vi "RSZVB Send Channel Trigger and Wait for OPC.vi"(8 "error in (no error)":errorcluster, 9 "Timeout (15000)":i32=15000, 10 "Channel (1)":i32=1, 11 "VISA session":refnum<visa-resource-name>) -> (0 "error out":errorcluster {"code" format="%.0x"}, 3 "dup VISA session":refnum<visa-resource-name>)   [LabVIEW 2015]
doc: "This VI starts a new single sweep sequence and waits for operation completed (OPC) before returning the status code. This function is available in single sweep mode only (INITiate<Ch>:CONTinuous OFF).\n\nNote(s):\n\n(1) In contrast to all other functions of the analyzer, INITiate<Ch>[:IMMediate] has been implemented to prevent overlapped execution.\n\n(2) The data of the last sweep can be read using CALCulate<Ch>:DATA:NSWeep? SDATa, <history_count>.\n\nRemote-control command(s):\nINITiate<Ch>[:IMMediate]\n*OPC?"
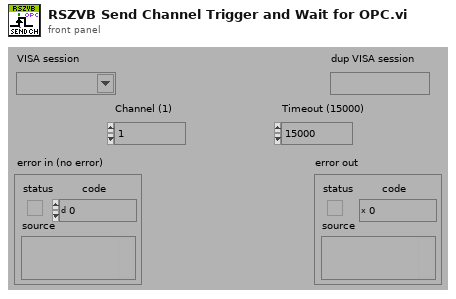
[diagram p1: front panel]
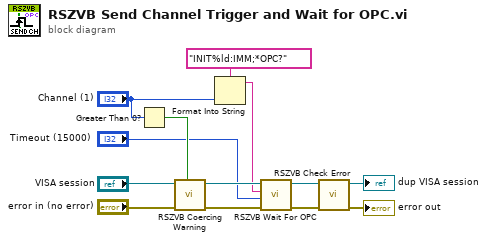
[diagram p0: block diagram]
diagram:
  n1 = Greater Than 0?(x="Channel (1)") -> (x > 0?=w6:bool)
  n2 = call "RSZVB Coercing Warning.vi"("In Range?"=w6, "error in (no error)"="error in (no error)", "VISA session"="VISA session") -> ("error out"=w9:errorcluster, "dup VISA session"=w10:refnum<visa-resource-name>)  [unwired: 7 in]
  n3 = Format Into String(format string="INIT%ld:IMM;*OPC?", "Channel (1)") -> (resulting string=w8:string)  [unwired: 2 in, 1 out]
  n4 = call "RSZVB Wait For OPC.vi"("error in (no error)"=w9, "Timeout (300000 ms)"="Timeout (15000)", "Command"=w8, "VISA session"=w10) -> ("error out"=w12:errorcluster, "dup VISA session"=w11:refnum<visa-resource-name>)  [unwired: 5 in, 1 out]
  n5 = call "RSZVB Check Error.vi"("error in (no error)"=w12, "VISA session"=w11) -> ("error out"=→"error out":errorcluster, "dup VISA session"=→"dup VISA session":refnum<visa-resource-name>)  [unwired: 8 in]
